vi "Moving_Average.vi"(2 "Sensor Value":dbl, 4 "FIFO-Size":i32=10) -> (6 "Moving Average":dbl=0.5633058732714724 caption="Mittelwert" format="%#.1f")   [LabVIEW 2012]
uses:
  <vilib>/Analysis/baseanly.llb/Mean (DBL).vi
  <vilib>/Analysis/NI_AALBase.lvlib
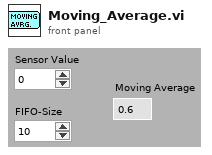
[diagram p1: front panel]
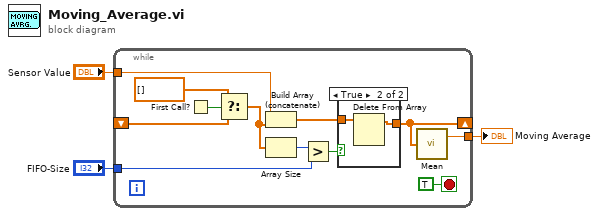
[diagram p0: block diagram]
diagram:
  n1 = while {
    shift-right: [w15] -> _
    shift-left: _ -> [w9]
    tunnel: [w6] -> w3
    tunnel: "Sensor Value" -> [w5]
    tunnel: "FIFO-Size" -> [w4]
    stop <- TRUE stop-if-true
    n2 = First Call?() -> (First Call?: T/F=w11:bool)
    n3 = Select(t=dbl[] [], s=w11, f=w9) -> (s? t:f=w8:dbl[])
    n4 = Build Array (concatenate)(w5, w8) -> (w12:dbl[])
    n5 = Array Size(array=w8) -> (size(s)=w14:i32)
    n6 = Greater?(x=w14, y=w4) -> (0:w13:bool)
    n7 = case shown="True" w13 {
      tunnel: [w16 w17] -> w15
      tunnel: w12 -> [w16 w18]
      frame False {
      }
      frame True {
        n8 = Delete From Array(array=w18) -> (array with subset deleted=w17:dbl[])  [unwired: 2 in, 1 out]
      }
    }
    n9 = call-poly <vilib>:"Mean.vi"("X"=w15) -> ("mean"=w6:dbl)  [unwired: 1 out]
  }
  "Moving Average" <- w3
